vi "Write State.vi"(8 "error in":errorcluster, 10 "State":bool, 11 "Change Filter State in":refnum<class "Change Filter State.lvclass">) -> (0 "error out":errorcluster, 3 "Change Filter State out":refnum<class "Change Filter State.lvclass">)   [LabVIEW 2014, in "eCRDS Library.lvlib" / "Change Filter State.lvclass"]
uses:
  Change Filter State.lvclass
  Change Filter State.lvclass/Change Filter State.ctl
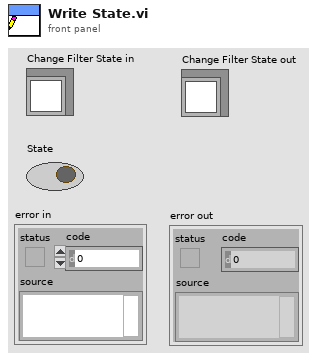
[diagram p1: front panel]
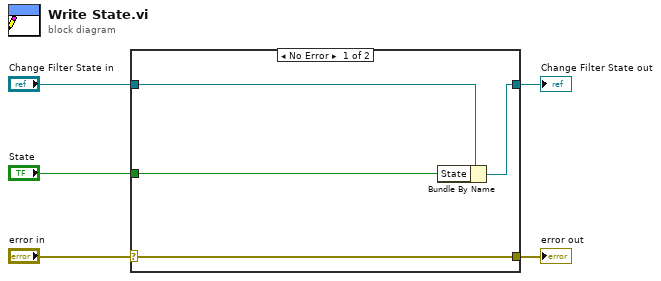
[diagram p0: block diagram]
diagram:
  n1 = case shown="No Error" "error in" {
    selector: "error in" -> [w9 w10]
    tunnel: [w9 w10] -> w4
    tunnel: [w7 w11] -> w2
    tunnel: "Change Filter State in" -> [w8 w11]
    tunnel: "State" -> [w6 _]
    frame No Error {
      n2 = Bundle By Name(cluster=w8, "State"=w6) -> (w7:refnum<class "Change Filter State.lvclass">)
    }
    frame Error {
    }
  }
  "error out" <- w4
  "Change Filter State out" <- w2
